vi "_Read_D.vi"(8 "error in (no error)":errorcluster, 11 "Postgres Connector In":refnum<class "Postgres Connector.lvclass">) -> (0 "error out":errorcluster, 3 "Postgres Connector Out":refnum<class "Postgres Connector.lvclass">)   [LabVIEW 2020, in "Postgres Connector.lvclass"]
doc: "This VI decode the \"D\" section of the message sent by the database and return the value of each rows."
uses:
  Postgres Connector.lvclass
  Enum_RowDescription_State_Machine.ctl
  Cluster_Reader_Infos.ctl
  Postgres Connector.lvclass/Postgres Connector.ctl
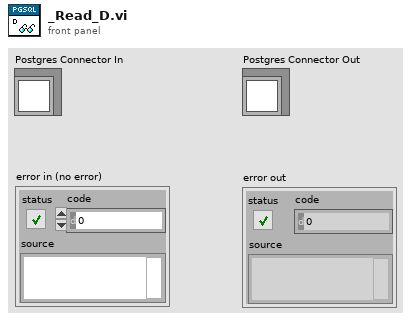
[diagram p1: front panel]
types:
  T1 = typedef "Postgres Connector.lvclass/Cluster_Reader_Infos.ctl" = cluster{"Byte Length":i32}
  T2 = typedef "Postgres Connector.lvclass/Enum_RowDescription_State_Machine.ctl" = enum16{"Check For Error", "Wait For T", "Wait For D", "Wait For Z", "C Byte Length", "Z Byte Length", "n Byte Length", "Byte Length", "Get Infos", "Check For End", "Flush", "Quit"}
  T3 = enum16{"Standard", "Buffered", "CRLF", "Immediate"}
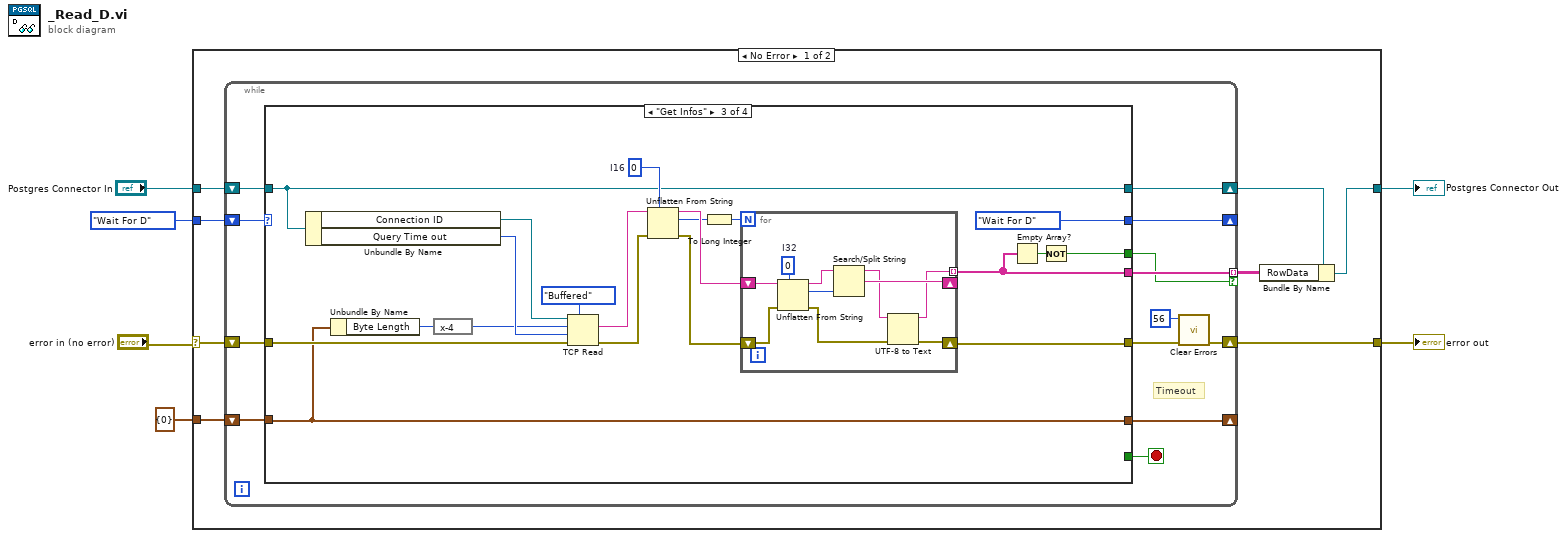
[diagram p0: block diagram]
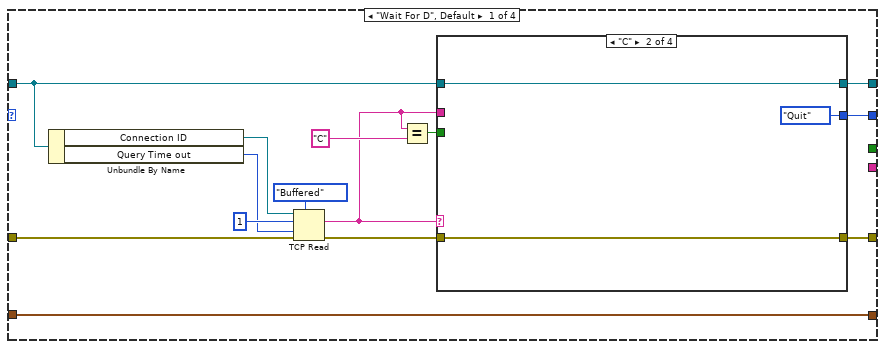
[diagram p2: hidden frame]
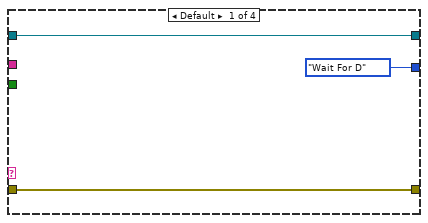
[diagram p3: hidden frame]
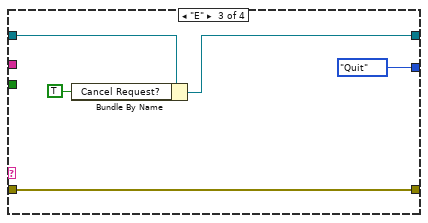
[diagram p4: hidden frame]
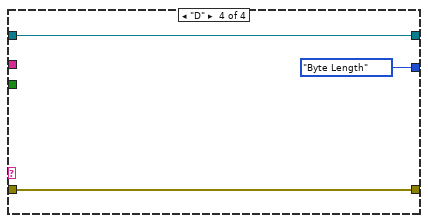
[diagram p5: hidden frame]
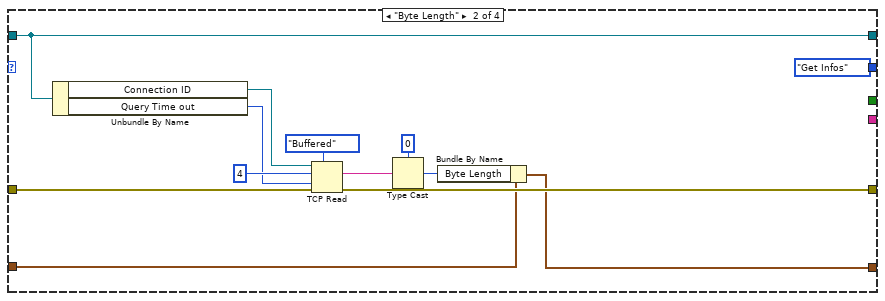
[diagram p6: hidden frame]
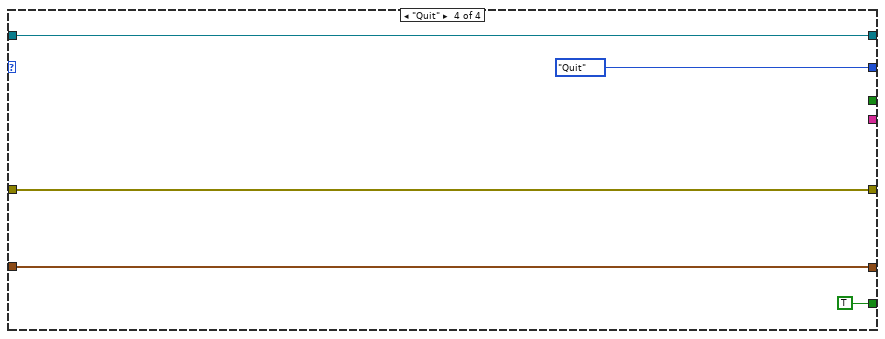
[diagram p7: hidden frame]
diagram:
  n1 = case shown="No Error" "error in (no error)" {
    selector: "error in (no error)" -> [w14 w105]
    tunnel: "Postgres Connector In" -> [w10 w104]
    tunnel: Enum_RowDescription_State_Machine."Wait For D" -> [w13 _]
    tunnel: [w12 w105] -> w3
    tunnel: T1 {"Byte Length"=0} ("Reader_Infos") -> [w11 _]
    tunnel: [w8 w104] -> w1
    frame No Error {
      n2 = while {
        shift-right: [w23] -> w12
        shift-left: w14 -> [w26]
        shift-right: [w21] -> _
        shift-left: w13 -> [w25]
        shift-right: [w19] -> _
        shift-left: w11 -> [w20]
        tunnel: [w17] -> w9 mode=indexing if=w16
        shift-right: [w15] -> w7
        shift-left: w10 -> [w27]
        stop <- w18 stop-if-true
        # "Timeout"
        n3 = case shown="\"Get Infos\"" w25 {
          tunnel: w27 -> [w33 w65 w69 w99]
          tunnel: w26 -> [w31 w64 w86 w102]
          tunnel: [w29 w63 w74 w102] -> w24
          tunnel: [w38 Enum_RowDescription_State_Machine."Get Infos" Enum_RowDescription_State_Machine."Wait For D" Enum_RowDescription_State_Machine."Quit"] -> w21
          tunnel: w20 -> [w37 w61 w85 w103]
          tunnel: [w37 w60 w85 w103] -> w19
          tunnel: [_ _ _ TRUE] -> w18
          tunnel: [_ _ w78 _] -> w17
          tunnel: [_ _ w82 _] -> w16
          tunnel: [w32 w65 w69 w99] -> w15
          frame "Wait For D", Default {
            n4 = Unbundle By Name(w33) -> ("Connection ID"=w40:refnum<k5>, "Query Time out"=w34:i32)
            n5 = TCP Read(connection ID=w40, bytes to read=1, error in (no error)=w31, 7:T3."Buffered" ("mode (standard)"), 9:w34) -> (data out=w28:string, error out=w30:errorcluster)  [unwired: 1 out]
            n6 = Equal?(x=w28, y="C") -> (x = y?=w35:bool)
            n7 = case shown="\"C\"" w28 {
              tunnel: [Enum_RowDescription_State_Machine."Wait For D" Enum_RowDescription_State_Machine."Quit" Enum_RowDescription_State_Machine."Quit" Enum_RowDescription_State_Machine."Byte Length"] -> w38
              tunnel: w35 -> [_ _ _ _]
              tunnel: w28 -> [_ _ _ _]
              tunnel: w33 -> [w44 w46 w51 w55]
              tunnel: [w44 w46 w50 w55] -> w32
              tunnel: w30 -> [w42 w47 w49 w53]
              tunnel: [w42 w47 w49 w53] -> w29
              frame Default {
              }
              frame "C" {
              }
              frame "E" {
                n8 = Bundle By Name(cluster=w51, "Cancel Request?"=TRUE) -> (w50:refnum<class "Postgres Connector.lvclass">)
              }
              frame "D" {
              }
            }
          }
          frame "Byte Length" {
            n9 = Unbundle By Name(w65) -> ("Connection ID"=w67:refnum<k5>, "Query Time out"=w56:i32)
            n10 = TCP Read(connection ID=w67, bytes to read=4, error in (no error)=w64, 7:T3."Buffered" ("mode (standard)"), 9:w56) -> (data out=w58:string, error out=w63:errorcluster)  [unwired: 1 out]
            n11 = Type Cast(type=0, x=w58) -> (*(type *) &x=w57:i32)
            n12 = Bundle By Name(cluster=w61, "Byte Length"=w57) -> (w60:T1)
          }
          frame "Get Infos" {
            w81 = i16 0  # I16
            n13 = Unbundle By Name(w69) -> ("Connection ID"=w87:refnum<k5>, "Query Time out"=w75:i32)
            n14 = Unbundle By Name(w85) -> ("Byte Length"=w71:i32)
            n15 = expression code="x-4"(w71) -> (w70:i32)
            n16 = TCP Read(connection ID=w87, bytes to read=w70, error in (no error)=w86, 7:T3."Buffered" ("mode (standard)"), 9:w75) -> (data out=w80:string, error out=w73:errorcluster)  [unwired: 1 out]
            n17 = Unflatten From String(type=w81, binary string=w80, error in (no error)=w73) -> (rest of the binary string=w79:string, value=w77:i16, error out=w72:errorcluster)  [unwired: 2 in]
            n18 = To Long Integer(number=w77) -> (32bit integer=w76:i32)
            n19 = for {
              N: w76 -> [_]
              tunnel: [w91] -> w78 mode=indexing
              shift-right: [w94] -> _
              shift-left: w79 -> [w97]
              shift-right: [w89] -> w74
              shift-left: w72 -> [w93]
              w98 = 0  # I32
              n20 = Unflatten From String(type=w98, binary string=w97, error in (no error)=w93) -> (rest of the binary string=w95:string, value=w96:i32, error out=w90:errorcluster)  [unwired: 2 in]
              n21 = Search/Split String(string=w95, offset (0)=w96) -> (substring before match=w92:string, match + rest of string=w94:string)  [unwired: 1 in, 1 out]
              n22 = UTF-8 to Text(8:w90, 11:w92) -> (0:w89:errorcluster, 3:w91:string)  [unwired: 1 in]
            }
            n23 = Empty Array?(array=w78) -> (empty?=w83:bool)
            n24 = Not(x=w83) -> (.not. x?=w82:bool)
          }
          frame "Quit" {
          }
        }
        n25 = call <vilib>:"Clear Errors.vi"("error in (no error)"=w24, "specific error code to clear (0: all)"=56) -> ("error out"=w23:errorcluster)  [unwired: 4 in, 1 out]
      }
      n26 = Bundle By Name(cluster=w7, "RowData"=w9) -> (w8:refnum<class "Postgres Connector.lvclass">)
    }
    frame Error {
    }
  }
  "error out" <- w3
  "Postgres Connector Out" <- w1
